vi "Set Inline Buffer.vi"(8 "error in (no error)":errorcluster, 9 "size":u64, 10 "address":u64, 11 "Plugin Interface in":refnum<class "Plugin Interface.lvclass">) -> (0 "error out":errorcluster, 3 "Plugin Interface out":refnum<class "Plugin Interface.lvclass">)   [LabVIEW 2017, in "DSF Core.lvlib" / "Plugin Interface.lvclass"]
uses:
  Plugin Interface.lvclass
  C:/Git/DSF/Data Sharing Framework/Source/Core/Engine/Classes/Interfaces/Interface/Interface.lvclass
  Command Data.ctl
  Command.ctl
  Command Parameters.ctl
  Interface/Interface.lvclass/Interface.ctl
  Write Plugin Command.vi
  Interface/Write Command.vi
  Interface/Write RT FIFO.vi
  Class Name.vi
  Interface/Errors.vi
  Dispatcher/Command Timeout.vi
  Read Plugin Response.vi
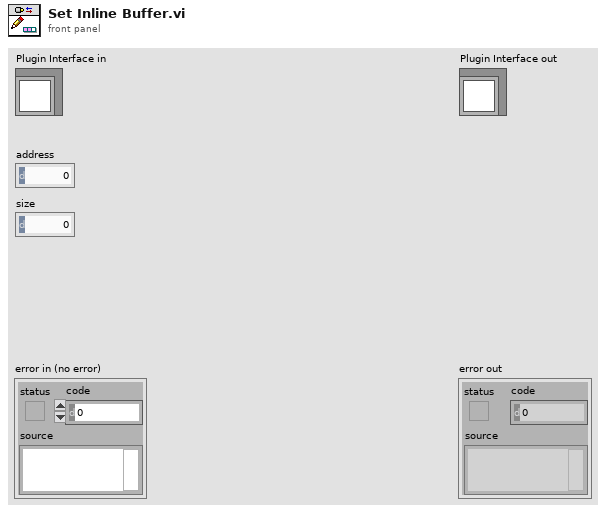
[diagram p1: front panel]
types:
  T1 = typedef "DSF Core.lvlib/Plugin Interface.lvclass/Command.ctl" = enum8{"Set Inline Buffer", "Rx", "Tx", "Shutdown"}
  T2 = typedef "DSF Core.lvlib/Plugin Interface.lvclass/Command Parameters.ctl" = cluster{"arg1":u64, "arg2":u64}
  T3 = typedef "DSF Core.lvlib/Plugin Interface.lvclass/Command Data.ctl" = cluster{"Command":T1, "Parameters":T2}
  T4 = typedef "DSF Core.lvlib/Plugin Interface.lvclass/Response Data.ctl" = cluster{"Response":T5, "Parameters":T6}
  T5 = typedef "DSF Core.lvlib/Plugin Interface.lvclass/Response.ctl" = enum8{"General Ack", "Shutting Down"}
  T6 = typedef "DSF Core.lvlib/Plugin Interface.lvclass/Response Parameters.ctl" = cluster{"arg1":u64, "arg2":u64}
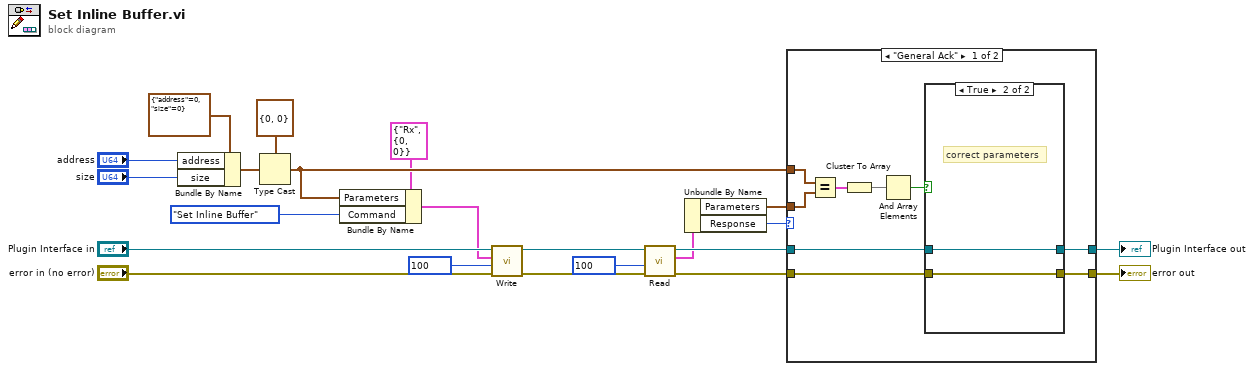
[diagram p0: block diagram]
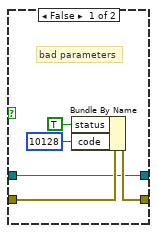
[diagram p2: hidden frame]
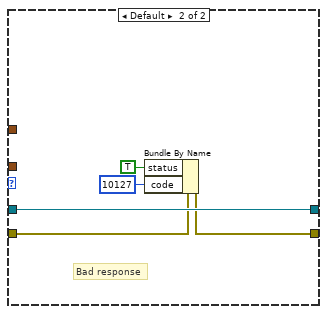
[diagram p3: hidden frame]
diagram:
  n1 = Bundle By Name(cluster=cluster{"address":u64, "size":u64} {"address"=0, "size"=0}, "address"="address", "size"="size") -> (w20:cluster{"address":u64, "size":u64})
  n2 = Type Cast(type=T2 {"arg1"=0, "arg2"=0} ("Command Parameters"), x=w20) -> (*(type *) &x=w2:T2)
  n3 = Bundle By Name(cluster=T3 {"Command"=enum."Rx", "Parameters"={"arg1"=0, "arg2"=0}} ("command"), "Parameters"=w2, "Command"=Command."Set Inline Buffer") -> (w13:T3)
  n4 = call-poly "Write.vi"("error in (no error)"="error in (no error)", "timeout in ms (0)"=100, "command"=w13, "Plugin Interface in"="Plugin Interface in") -> ("error out"=w11:errorcluster, "Plugin Interface out"=w12:refnum<class "Plugin Interface.lvclass">)  [unwired: 6 in]
  n5 = call-poly "Read.vi"("error in (no error)"=w11, "timeout in ms (0)"=100, "Plugin Interface in"=w12) -> ("error out"=w7:errorcluster, "response"=w5:T4, "Plugin Interface out"=w9:refnum<class "Plugin Interface.lvclass">)  [unwired: 5 in, 1 out]
  n6 = Unbundle By Name(w5) -> ("Parameters"=w3:T6, "Response"=w4:T5)
  n7 = case shown="\"General Ack\"" w4 {
    tunnel: w9 -> [w29 w43]
    tunnel: [w27 w43] -> w8
    tunnel: w7 -> [w28 w40]
    tunnel: [w26 w39] -> w6
    tunnel: w3 -> [w31 _]
    tunnel: w2 -> [w30 _]
    frame "General Ack" {
      n8 = Equal?(x=w30, y=w31) -> (x = y?=w25:cluster{"arg1":bool, "arg2":bool})
      n9 = Cluster To Array(cluster=w25) -> (array=w24:bool[])
      n10 = And Array Elements(Boolean array=w24) -> (logical AND=w23:bool)
      n11 = case shown="True" w23 {
        tunnel: w29 -> [w32 w38]
        tunnel: w28 -> [w34 w37]
        tunnel: [w32 w38] -> w27
        tunnel: [w33 w37] -> w26
        frame False {
          # "bad parameters"
          n12 = Bundle By Name(cluster=w34, "status"=TRUE, "code"=10128) -> (w33:errorcluster)
        }
        frame True {
          # "correct parameters"
        }
      }
    }
    frame Default {
      # "Bad response"
      n13 = Bundle By Name(cluster=w40, "status"=TRUE, "code"=10127) -> (w39:errorcluster)
    }
  }
  "error out" <- w6
  "Plugin Interface out" <- w8
